vi "Simple MQTT Broker.vi"() -> ()   [LabVIEW 2020, in "MQTT_Client.lvlib"]
doc: "A Simple MQTT Broker by PantherLAB\nAugust 2021\nCLA Enrique Noé Arias"
uses:
  MQTT_Client.lvlib
  <vilib>/LabVIEW Open Source Project/OpenSerializer JKI JSON/Serializer.JSON.lvclass
  C:/Program Files (x86)/National Instruments/LabVIEW 2020/vi.lib/LabVIEW Open Source Project/OpenSerializer/Serializer/Serializer.lvclass
  <vilib>/LabVIEW Open Source Project/MQTT Connection/MQTT_Base/Base Class/MQTT_Base.lvclass/MQTT_Base.ctl
  <vilib>/G Open Source Project for LabVIEW/MQTT Broker/Server class/Server.lvclass/Server.ctl
  <vilib>/LabVIEW Open Source Project/MQTT Control Packets/Control Packets/ControlPacket/ControlPacket.lvclass/ControlPacket.ctl
  <vilib>/LabVIEW Open Source Project/MQTT TCP Connection/MQTT_TCP/Connection/TCPConnection.lvclass
  C:/Program Files (x86)/National Instruments/LabVIEW 2020/vi.lib/LabVIEW Open Source Project/MQTT Connection/MQTT_Connection/Connection/Connection.lvclass
  <vilib>/G Open Source Project for LabVIEW/MQTT Broker/Server class/Server.lvclass
  C:/Program Files (x86)/National Instruments/LabVIEW 2020/vi.lib/LabVIEW Open Source Project/MQTT Connection/MQTT_Base/Base Class/MQTT_Base.lvclass
  <vilib>/LabVIEW Open Source Project/OpenSerializer/Serializer.FlattenedString/Serializer.FlattenedString.lvclass
  <vilib>/LabVIEW Open Source Project/MQTT Control Packets/Control Packets/PUBLISH/PUBLISH.lvclass
  C:/Program Files (x86)/National Instruments/LabVIEW 2020/vi.lib/LabVIEW Open Source Project/MQTT Control Packets/Control Packets/ControlPacket/ControlPacket.lvclass
  <vilib>/LabVIEW Open Source Project/OpenSerializer/Serializer/Serializer.lvclass
  <vilib>/LabVIEW Open Source Project/MQTT Connection/MQTT_Base/Base Class/MQTT_Base.lvclass
  <vilib>/LabVIEW Open Source Project/MQTT Control Packets/Control Packets/ControlPacket/ControlPacket.lvclass
panel:
  out "Last Message":string
  out "Who is Publishing--Topic":string
  out "Port":u16=1883
  out "MQTT Broker":string
  out "Clients\nConnected":u32
  out "error server":errorcluster
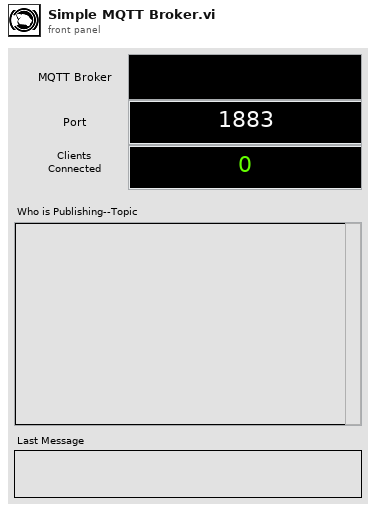
[diagram p1: front panel]
types:
  T1 = typedef "MQTT Server.lvlib/Server.lvclass/Public Events -- cluster.ctl" = cluster{"NbConnections":refnum<user-event>}
  T2 = typedef "MQTT Base.lvlib/MQTT_Base.lvclass/Public Events -- cluster.ctl" = cluster{"Stop Event":refnum<user-event>, "Error Event":refnum<user-event>, "Inbound Message":refnum<user-event>}
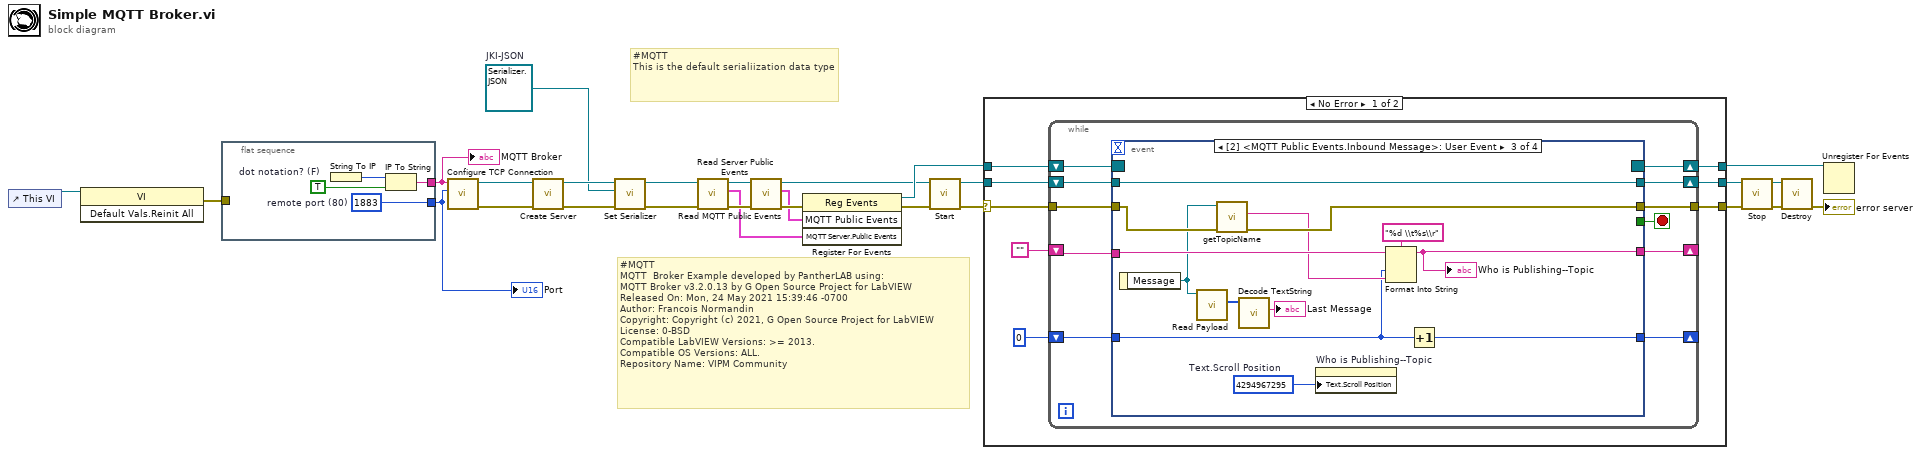
[diagram p0: block diagram]
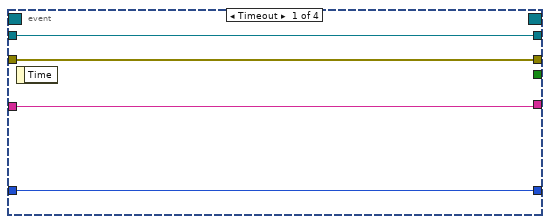
[diagram p2: hidden frame]
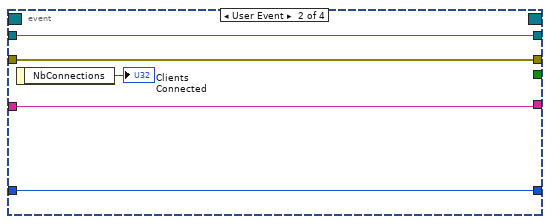
[diagram p3: hidden frame]
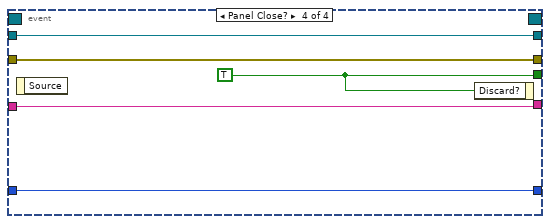
[diagram p4: hidden frame]
diagram:
  w1 = refnum<class "Serializer.JSON.lvclass"> refnum  # JKI-JSON
  # "#MQTT \nMQTT  Broker Example developed by PantherLAB using:\nMQTT Broker v3.2.0.13 by G Open Source Project for LabVIEW\nReleased On: Mon, 24 May 2021 15:39:46 -0700\nAuthor: Francois Normandin\nCopyright: Copyright (c) 2021, G Open Source Project for LabVIEW\nLicense: 0-BSD\nCompatible LabVIEW Versions: >= 2013.\nCompatible OS Versions: ALL.\nRepository Name: VIPM Community"
  # "#MQTT\nThis is the default serialiization data type"
  n1 = control-ref of="This VI"() -> (w2:refnum<vi>)
  n2 = invoke class="VI" method="Default Vals.Reinit All"(reference=w2) -> (error out=w17:errorcluster)  [unwired: 2 in, 2 out]
  n3 = flat-sequence {
    tunnel: [w29] -> w10
    tunnel: [w28] -> w9
    tunnel: w17 -> [_]
    frame #0 {
      w28 = u16 1883  # remote port (80)
      w31 = TRUE  # dot notation? (F)
      n4 = String To IP() -> (0:w30:u32)  [unwired: 1 in]
      n5 = IP To String(1:w31, 2:w30) -> (0:w29:string)
    }
  }
  n6 = call <vilib>:"Configure TCP Connection.vi"("remote port (80)"=w9, "address (localhost)"=w10) -> ("error out"=w21:errorcluster, "TCPConnection"=w11:refnum<class "TCPConnection.lvclass">)  [unwired: 8 in]
  n7 = call <vilib>:"Create Server.vi"("error in (no error)"=w21, "Connection Configuration"=w11) -> ("error out"=w22:errorcluster, "Server"=w4:refnum<class "Server.lvclass">)  [unwired: 8 in]
  n8 = call <vilib>:"Set Serializer.vi"("error in (no error)"=w22, "Serializer (default: Flattened String)"=w1, "MQTT_Base"=w4) -> ("error out"=w18:errorcluster, "MQTT_Base out"=w3:refnum<class "Server.lvclass">)  [unwired: 7 in]
  n9 = call <vilib>:"Read Server Public Events.vi"("error in (no error)"=w18, "Server in"=w3) -> ("error out"=w20:errorcluster, "MQTT Server.Public Events"=w5:T1, "Server out"=w8:refnum<class "Server.lvclass">)  [unwired: 7 in]
  n10 = call <vilib>:"Read MQTT Public Events.vi"("error in (no error)"=w20, "MQTT_Base in"=w8) -> ("error out"=w19:errorcluster, "MQTT Public Events"=w6:T2, "MQTT_Base out"=w7:refnum<class "Server.lvclass">)  [unwired: 7 in]
  n11 = register-events(error in=w19, w6, w5) -> (reference out=w12:refnum<event-registration>, error out=w23:errorcluster)  [unwired: 1 in]
  n12 = call <vilib>:"Start.vi"("error in (no error)"=w23, "MQTT_Base in"=w7) -> ("error out"=w24:errorcluster, "MQTT_Base out"=w14:refnum<class "Server.lvclass">)  [unwired: 7 in, 1 out]
  n13 = case shown="No Error" w24 {
    selector: w24 -> [w38 w80]
    tunnel: w14 -> [w37 w79]
    tunnel: [w36 w79] -> w16
    tunnel: w12 -> [w35 w78]
    tunnel: [w34 w78] -> w13
    tunnel: [w39 w80] -> w27
    frame No Error {
      n14 = while {
        shift-right: [w46] -> w36
        shift-left: w37 -> [w48]
        tunnel: [w50] -> w39
        tunnel: w38 -> [w49]
        shift-right: [w44] -> w34
        shift-left: w35 -> [w45]
        shift-right: [w41] -> _
        shift-left: "" -> [w43]
        shift-right: [w40] -> _
        shift-left: 0 -> [w42]
        stop <- w47 stop-if-true
        n15 = event shown="[2] <MQTT Public Events.Inbound Message>: User Event" {
          selector: w45 -> [_ _ _ _]
          dyn-events: [_ _ _ _] -> w44
          timeout: _ -> [_ _ _ _]
          tunnel: w48 -> [w53 w58 w64 w76]
          tunnel: [_ _ _ w75] -> w47
          tunnel: [w53 w58 w64 w76] -> w46
          tunnel: [w54 w59 w72 w77] -> w50
          tunnel: w49 -> [w54 w59 w71 w77]
          tunnel: w43 -> [w52 w56 w70 w74]
          tunnel: w42 -> [w51 w55 w67 w73]
          tunnel: [w52 w56 w68 w74] -> w41
          tunnel: [w51 w55 w66 w73] -> w40
          event Timeout {
            n16 = event-data() -> ()  [unwired: 1 in, 1 out]
          }
          event User Event {
            n17 = event-data() -> ("NbConnections"=→"Clients\nConnected":u32)  [unwired: 1 in]
          }
          event User Event {
            w65 = u32 4294967295  # Text.Scroll Position
            n18 = event-data() -> ("Message"=w60:refnum<class "PUBLISH.lvclass">)  [unwired: 1 in]
            n19 = call <vilib>:"Read Payload.vi"("ControlPacket in"=w60) -> ("Payload"=w63:u8[])  [unwired: 9 in, 1 out]
            n20 = call <vilib>:"getTopicName.vi"("error in (no error)"=w71, "PUBLISH in"=w60) -> ("error out"=w72:errorcluster, "Topic"=w69:string)  [unwired: 7 in, 1 out]
            n21 = call <vilib>:"Decode TextString.vi"("Length-Prefixed Field"=w63) -> ("Text String"=→"Last Message":string)  [unwired: 8 in, 2 out]
            n22 = property on="Who is Publishing--Topic" class="Str"("Text.Scroll Position"=w65) -> ()  [unwired: 2 in, 2 out]
            n23 = Format Into String(format string="%d \\t%s\\r", initial string=w70, w67, w69) -> (resulting string=w68:string)  [unwired: 1 in, 1 out]
            "Who is Publishing--Topic" <- w68
            n24 = Increment(x=w67) -> (x+1=w66:i32)
          }
          event Panel Close? {
            w75 = TRUE ("Discard?")
            n25 = event-data() -> ()  [unwired: 1 in, 1 out]
            n26 = event-data("Discard?"=w75) -> ()  [unwired: 1 in, 1 out]
          }
        }
      }
    }
    frame Error {
    }
  }
  n27 = call <vilib>:"Stop.vi"("error in (no error)"=w27, "MQTT_Base in"=w16) -> ("error out"=w26:errorcluster, "MQTT_Base out"=w15:refnum<class "Server.lvclass">)  [unwired: 7 in, 1 out]
  n28 = call <vilib>:"Destroy.vi"("error in (no error)"=w26, "MQTT_Base in"=w15) -> ("error out"=→"error server":errorcluster)  [unwired: 8 in, 1 out]
  n29 = Unregister For Events(event registration refnum=w13) -> ()  [unwired: 1 in, 1 out]
  "MQTT Broker" <- w10
  "Port" <- w9
